vi "Close Hardware Session.vi"(8 "error in":errorcluster, 11 "hardware handles":T1) -> (0 "error out":errorcluster)   [LabVIEW 2020, in "Ballard ARINC 429 Engine.lvlib" / "Custom Device.lvlib"]
uses:
  Custom Device.lvlib
  <instrlib>/BTICardLib/BTICardLV.lvlib
  <instrlib>/BTI429Lib/BTI429LV.lvlib
  Hardware Handles.ctl
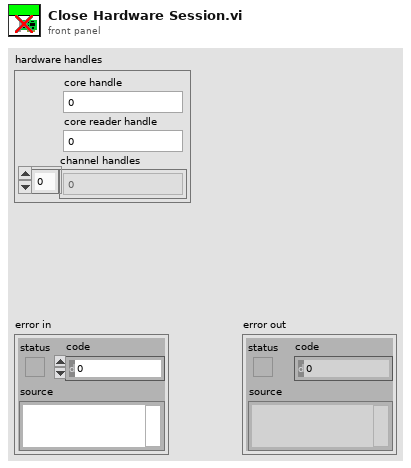
[diagram p1: front panel]
types:
  T1 = typedef "Ballard ARINC 429 Engine.lvlib/Custom Device.lvlib/Hardware Handles.ctl" = cluster{"core handle":u64, "core reader handle":u64, "channel handles":u64[]}
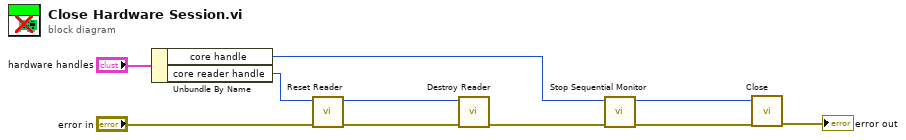
[diagram p0: block diagram]
diagram:
  n1 = Unbundle By Name("hardware handles") -> ("core handle"=w7:u64, "core reader handle"=w8:u64)
  n2 = call <instrlib>:"Reset Reader.vi"("error in (no error)"="error in", "reader handle in"=w8) -> ("error out"=w6:errorcluster, "reader handle out"=w4:u64)  [unwired: 8 in]
  n3 = call <instrlib>:"Destroy Reader.vi"("error in (no error)"=w6, "reader handle in"=w4) -> ("error out"=w5:errorcluster)  [unwired: 9 in]
  n4 = call <instrlib>:"Stop Sequential Monitor.vi"("error in (no error)"=w5, "core handle in"=w7) -> ("error out"=w9:errorcluster, "core handle out"=w10:u64)  [unwired: 8 in]
  n5 = call <instrlib>:"Close.vi"("error in (no error)"=w9, "core handle in"=w10) -> ("error out"=→"error out":errorcluster)  [unwired: 8 in, 1 out]
